vi "Unique Q Name.vi"() -> (3 "unique Q name":string)   [LabVIEW 2017]
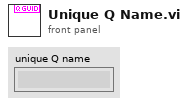
[diagram p1: front panel]
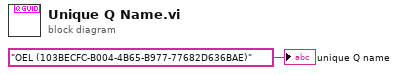
[diagram p0: block diagram]
diagram:
  "unique Q name" <- "OEL (103BECFC-B004-4B65-B977-77682D636BAE)" ("name (unnamed)")
